vi "Write Update Msg.vi"(10 "Update Msg.lvclass":refnum<class "Update Msg.lvclass">, 11 "Timing Engine in":refnum<class "Timing Engine.lvclass">) -> (3 "Timing Engine out":refnum<class "Timing Engine.lvclass">)   [LabVIEW 2017, in "Assert API Components.lvlib" / "Assert Display.lvlib" / "Timing Engine.lvlib" / "Timing Engine.lvclass"]
uses:
  Timing Engine.lvclass
  Timing Engine Messages/Update Msg/Update Msg.lvclass
  Timing Engine.lvclass/Timing Engine.ctl
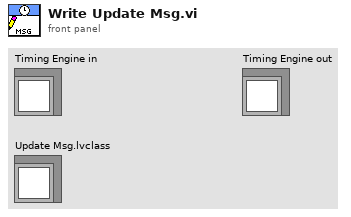
[diagram p1: front panel]
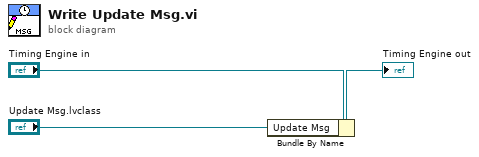
[diagram p0: block diagram]
diagram:
  n1 = Bundle By Name(cluster="Timing Engine in", "Update Msg"="Update Msg.lvclass") -> (→"Timing Engine out":refnum<class "Timing Engine.lvclass">)
